vi "Delete Experiment.vi"(3 "error in (no error)":errorcluster, 4 "Experiment to Delete":T1, 5 "Database.lvlib:Data Store.lvclass":refnum<class "Data Store.lvclass">) -> (0 "error out":errorcluster, 2 "Database.lvlib:Data Store.lvclass 2":refnum<class "Data Store.lvclass">)   [LabVIEW 2011, in "Database.lvlib" / "Data Store.lvclass"]
uses:
  Data Store.lvclass
  Experiment.ctl
  <vilib>/addons/database/Auxilliary.llb/DB Tools Transaction.ctl
  <vilib>/addons/database/Auxilliary.llb/DB Tools Isolation Level.ctl
  <vilib>/addons/database/Auxilliary.llb/DB Tools Parameter Info.ctl
  <vilib>/addons/database/Auxilliary.llb/DB Tools DataTypes.ctl
  <vilib>/addons/database/Auxilliary.llb/DB Tools Parameter Dir.ctl
  Data Store.lvclass/Data Store.ctl
  <vilib>/addons/database/Connection.llb/Conn Transaction.vi
  <vilib>/addons/database/Command.llb/Cmd Set Parameter Value (C).vi
  <vilib>/addons/database/Command.llb/Cmd Execute.vi
  <vilib>/addons/database/Recordset.llb/Rec Destroy - Command.vi
  <vilib>/addons/database/Command.llb/Cmd Delete.vi
  <vilib>/addons/database/NI_Database_API.lvlib
  Database.lvlib
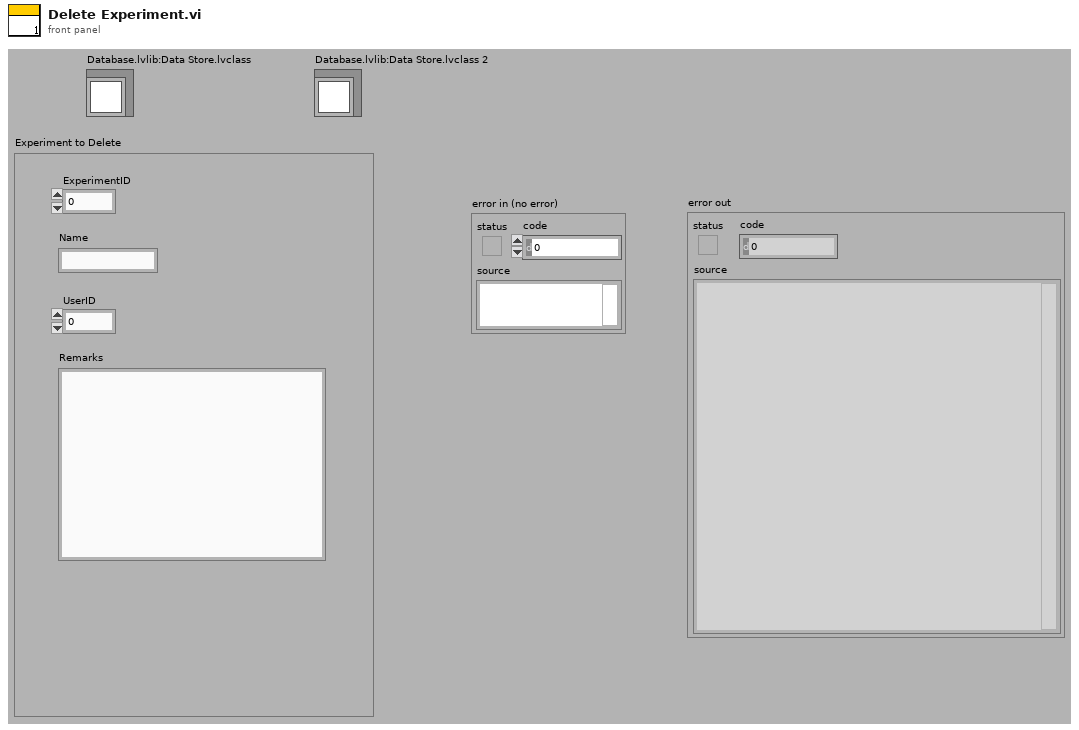
[diagram p1: front panel]
types:
  T1 = typedef "Database.lvlib/Experiment.ctl" = cluster{"ExperimentID":i32, "Name":string, "UserID":i32, "Remarks":string}
  T2 = typedef "NI_Database_API.lvlib/DB Tools Parameter Info.ctl" = cluster{"parameter name":string, "type":T3, "direction":T4, "value":variant}
  T3 = typedef "NI_Database_API.lvlib/DB Tools DataTypes.ctl" = enum16{"String", "Long (I32)", "Single (SGL)", "Double (DBL)", "Date/Time", "Binary"}
  T4 = typedef "NI_Database_API.lvlib/DB Tools Parameter Dir.ctl" = enum32{"Input", "Output", "Input/Output", "Return Value"}
  T5 = typedef "NI_Database_API.lvlib/DB Tools Isolation Level.ctl" = enum16{"chaos", "read uncommitted", "read committed", "repeatable read", "serializable"}
  T6 = typedef "NI_Database_API.lvlib/DB Tools Transaction.ctl" = enum16{"begin", "commit", "rollback"}
  T7 = typedef "NI_Database_API.lvlib/Conn ObjectReference.ctl" = refnum<k1>
  T8 = typedef "NI_Database_API.lvlib/Cmd ObjectReference.ctl" = refnum<k1>
  T9 = typedef "NI_Database_API.lvlib/Cmd-Rec Object Reference.ctl" = refnum<k1>
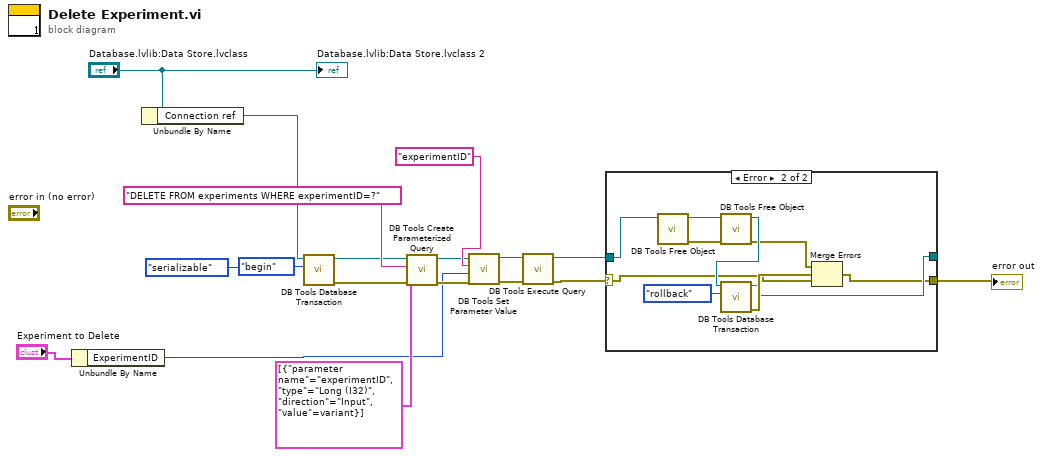
[diagram p0: block diagram]
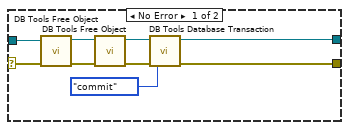
[diagram p2: hidden frame]
diagram:
  n1 = Unbundle By Name("Experiment to Delete") -> ("ExperimentID"=w7:i32)
  n2 = Unbundle By Name("Database.lvlib:Data Store.lvclass") -> ("Connection ref"=w15:T7)
  n3 = call-poly <vilib>:"DB Tools Database Transaction.vi"("isolation level (chaos)"=DB_Tools_Isolation_Level."serializable", "operation (begin)"=DB_Tools_Transaction."begin", "connection reference"=w15) -> ("error out"=w12:errorcluster, "connection reference out"=w11:T7)  [unwired: 3 in]
  n4 = call <vilib>:"DB Tools Create Parameterized Query.vi"("error in (no error)"=w12, "parameters"=T2[] [{"parameter name"="experimentID", "type"=enum."Long (I32)", "direction"=enum."Input", "value"=variant}], "SQL query"="DELETE FROM experiments WHERE experimentID=?", "connection reference"=w11) -> ("error out"=w10:errorcluster, "command reference"=w6:T8)  [unwired: 3 in, 1 out]
  n5 = call-poly <vilib>:"DB Tools Set Parameter Value.vi"("error in (no error)"=w10, "value"=w7, "parameter index"="experimentID", "command reference"=w6) -> ("error out"=w5:errorcluster, "command reference out"=w4:T8)  [unwired: 4 in]
  n6 = call-poly <vilib>:"DB Tools Execute Query.vi"("error in (no error)"=w5, "command reference"=w4) -> ("error out"=w3:errorcluster, "command-recordset reference"=w2:T9)  [unwired: 6 in]
  n7 = case shown="Error" w3 {
    selector: w3 -> [w27 w30]
    tunnel: w2 -> [w26 w37]
    tunnel: [w20 w28] -> w1
    tunnel: [w19 w29] -> _
    frame No Error {
      n8 = call-poly <vilib>:"DB Tools Free Object.vi"("error in (no error)"=w27, "command-recordset reference"=w26) -> ("error out"=w25:errorcluster, "command reference"=w24:T8)  [unwired: 8 in]
      n9 = call-poly <vilib>:"DB Tools Free Object.vi"("error in (no error)"=w25, "command reference"=w24) -> ("error out"=w23:errorcluster, "connection reference"=w22:T7)  [unwired: 8 in]
      n10 = call-poly <vilib>:"DB Tools Database Transaction.vi"("error in (no error)"=w23, "operation (begin)"=DB_Tools_Transaction."commit", "connection reference"=w22) -> ("error out"=w20:errorcluster, "connection reference out"=w19:T7)  [unwired: 3 in]
    }
    frame Error {
      n11 = call-poly <vilib>:"DB Tools Free Object.vi"("command-recordset reference"=w37) -> ("error out"=w33:errorcluster, "command reference"=w36:T8)  [unwired: 9 in]
      n12 = call-poly <vilib>:"DB Tools Free Object.vi"("error in (no error)"=w33, "command reference"=w36) -> ("error out"=w32:errorcluster, "connection reference"=w35:T7)  [unwired: 8 in]
      n13 = call-poly <vilib>:"DB Tools Database Transaction.vi"("operation (begin)"=DB_Tools_Transaction."rollback", "connection reference"=w35) -> ("error out"=w31:errorcluster, "connection reference out"=w29:T7)  [unwired: 4 in]
      n14 = Merge Errors(w32, w31, w30) -> (w28:errorcluster)
    }
  }
  "error out" <- w1
  "Database.lvlib:Data Store.lvclass 2" <- "Database.lvlib:Data Store.lvclass"
